vi "manage execution errors.vi"(8 "error in (no error)":errorcluster, 11 "Channel in":refnum<class "SPARC4_Channel.lvclass">) -> (0 "error out":errorcluster, 3 "Channel out":refnum<class "SPARC4_Channel.lvclass">)   [LabVIEW 2018, in "SPARC4_Channel.lvclass"]
uses:
  SPARC4_Channel.lvclass
  Log File/Log File.lvclass
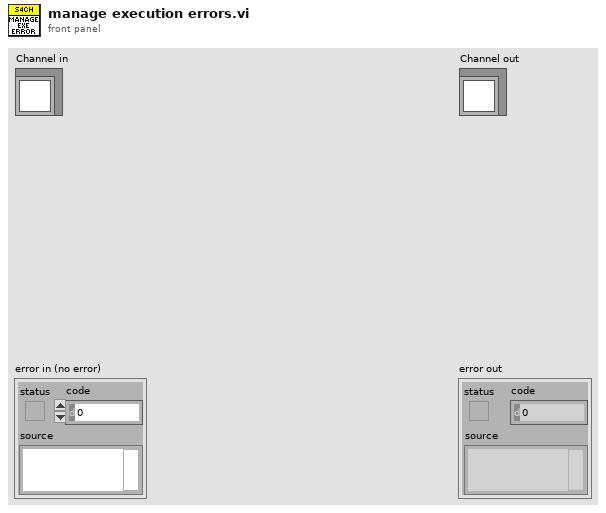
[diagram p1: front panel]
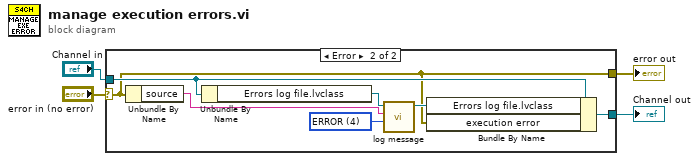
[diagram p0: block diagram]
diagram:
  n1 = case shown="Error" "error in (no error)" {
    selector: "error in (no error)" -> [w5 w7]
    tunnel: [w5 w7] -> w4
    tunnel: [w6 w8] -> w3
    tunnel: "Channel in" -> [w6 w13]
    frame No Error {
    }
    frame Error {
      w10 = u16 4 items=[" STATUS ", " DEBBUG ", "  INFO  ", "WARNING ", " ERROR  ", "CRITICAL"] ("log level")
      n2 = Unbundle By Name(w7) -> ("source"=w9:string)
      n3 = Unbundle By Name(w13) -> ("Errors log file.lvclass"=w12:refnum<class "Log File.lvclass">)
      n4 = call-dynamic "log message.vi"("log level"=w10, "Message to log"=w9, "Log File in"=w12) -> ("Log File out"=w11:refnum<class "Log File.lvclass">)  [unwired: 7 in, 1 out]
      n5 = Bundle By Name(cluster=w13, "Errors log file.lvclass"=w11, "execution error"=w7) -> (w8:refnum<class "SPARC4_Channel.lvclass">)
    }
  }
  "error out" <- w4
  "Channel out" <- w3
